vi "Create WebService.vi"() -> ()   [LabVIEW 2019, in "HTTP Server.lvlib"]
uses:
  HTTP Server.lvlib
  WebService reference.ctl
  Listener Information.ctl
panel:
  in  "WebService引用":T1={"IP Address"="127.0.0.1", "Port"=8003, "listener ID"=refnum}
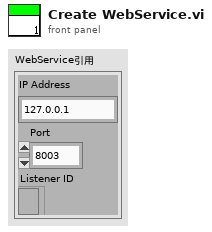
[diagram p1: front panel]
types:
  T1 = typedef "HTTP Server.lvlib/WebService reference.ctl" = cluster{"IP Address":string, "Port":u16, "listener ID":refnum<k5>}
  T2 = typedef "HTTP Server.lvlib/Listener Information.ctl" = cluster{"连接ID":refnum<k5>}
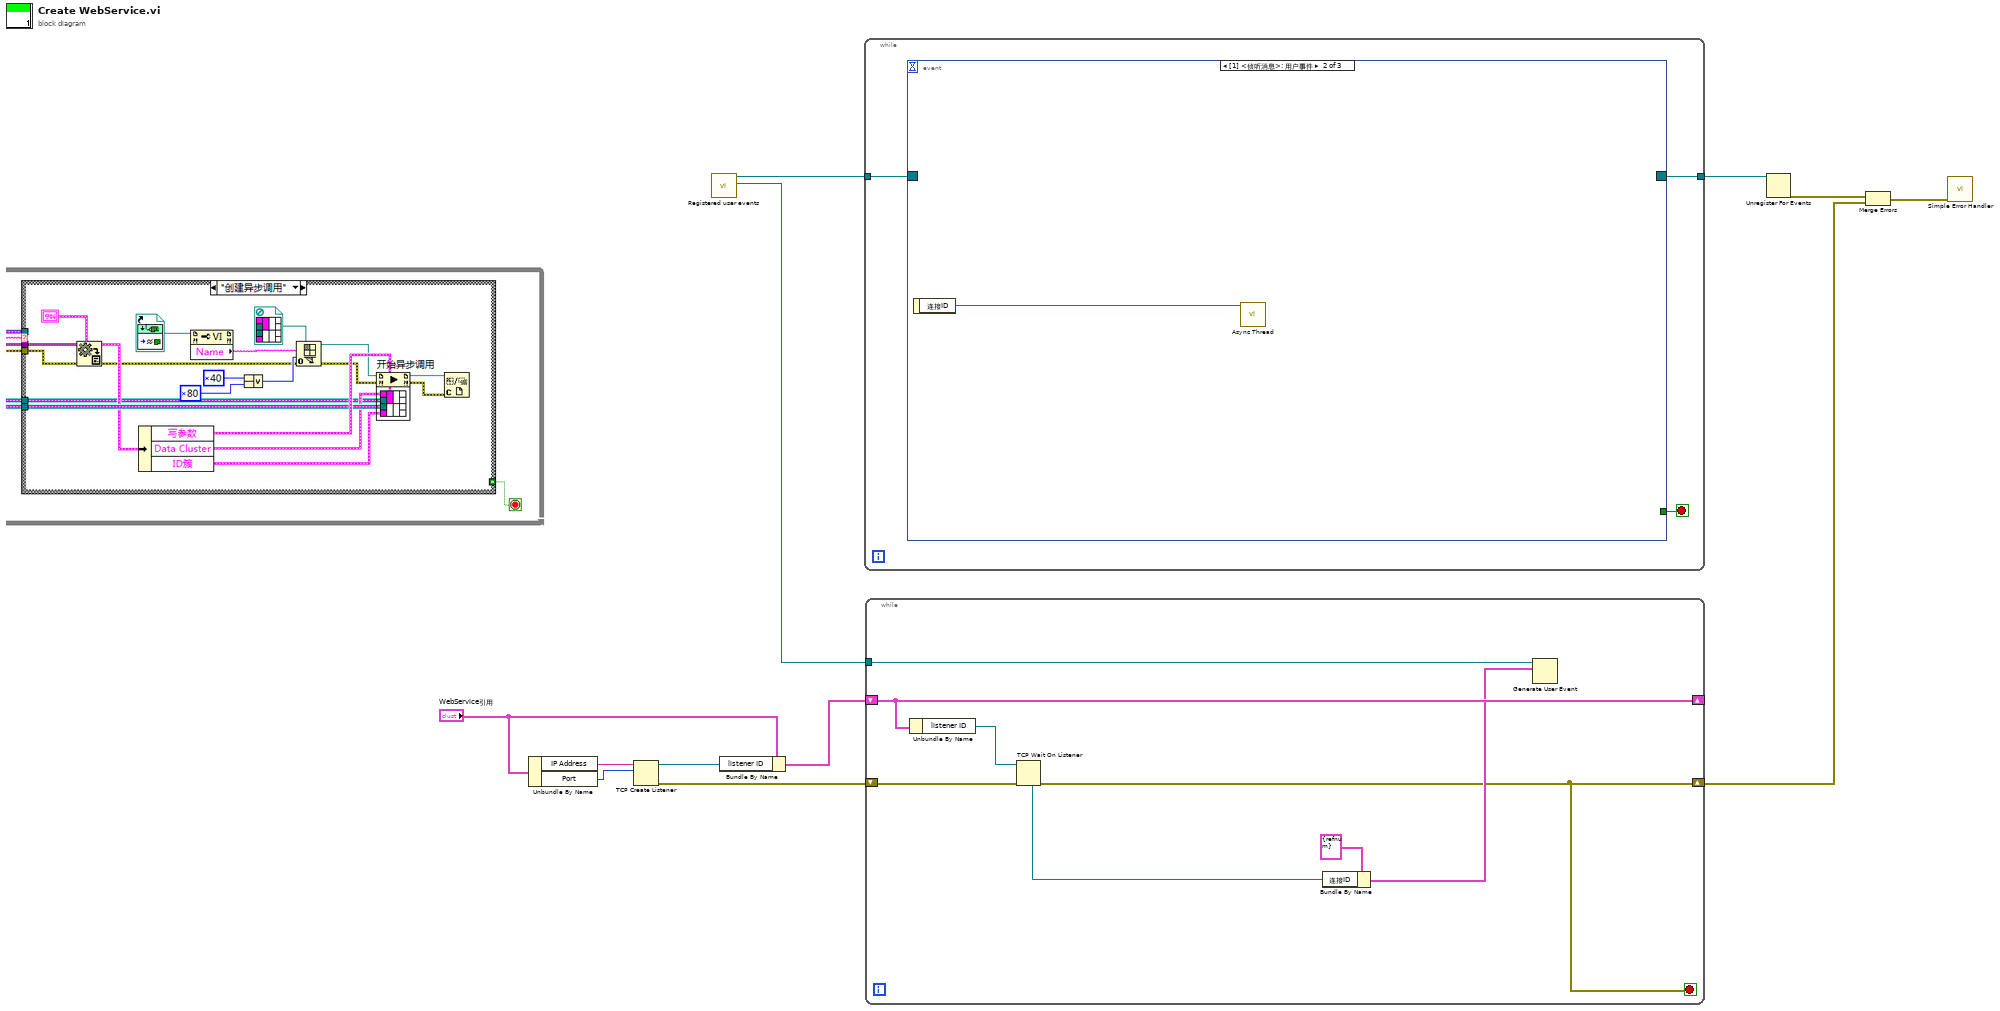
[diagram p0: block diagram]
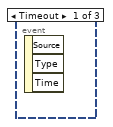
[diagram p2: hidden frame]
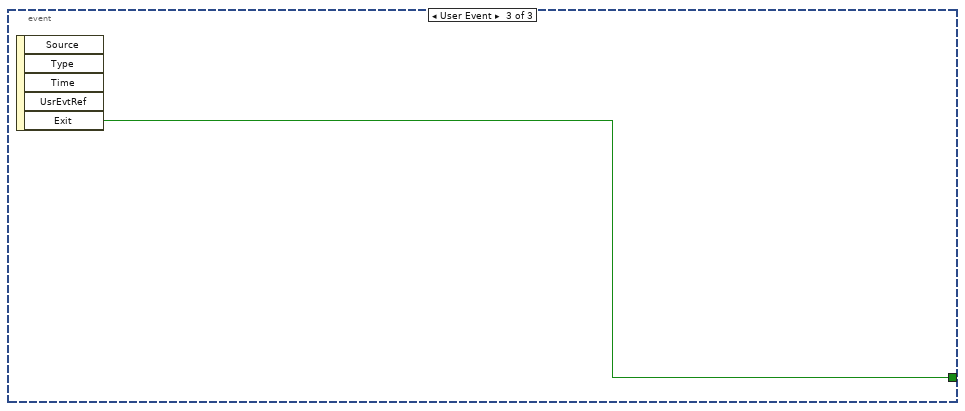
[diagram p3: hidden frame]
diagram:
  n1 = Unbundle By Name("WebService引用") -> ("IP Address"=w10:string, "Port"=w9:u16)
  n2 = TCP Create Listener(10:w9, 11:w10) -> (0:w5:errorcluster, 3:w7:refnum<k5>)  [unwired: 3 in, 1 out]
  n3 = call "Registered user events.vi"() -> ("用户事件输出_侦听消息"=w11:refnum<user-event>, "事件注册引用句柄"=w12:refnum<event-registration>)  [unwired: 9 in, 1 out]
  n4 = Bundle By Name(cluster="WebService引用", "listener ID"=w7) -> (w6:T1)
  n5 = while {
    tunnel: w12 -> [w15]
    tunnel: [w13] -> w4
    stop <- w14 stop-if-true
    n6 = event shown="[1] <侦听消息>: 用户事件" {
      selector: w15 -> [_ _ _]
      dyn-events: [_ _ _] -> w13
      timeout: _ -> [_ _ _]
      tunnel: [_ _ w17] -> w14
      event Timeout {
        n7 = event-data() -> ()  [unwired: 1 in, 3 out]
      }
      event User Event {
        n8 = event-data() -> ("连接ID"=w16:refnum<k5>)  [unwired: 1 in]
        n9 = call "Async Thread.vi"("TCP网络连接引用句柄"=w16) -> ()  [unwired: 11 in]
      }
      event User Event {
        n10 = event-data() -> ("Exit"=w17:bool)  [unwired: 1 in, 4 out]
      }
    }
  }
  n11 = while {
    tunnel: w11 -> [w25]
    shift-right: [w24] -> _
    shift-left: w6 -> [w24]
    shift-right: [w18] -> w2
    shift-left: w5 -> [w22]
    stop <- w18 stop-if-true
    n12 = Unbundle By Name(w24) -> ("listener ID"=w23:refnum<k5>)
    n13 = TCP Wait On Listener(8:w22, 11:w23) -> (0:w18:errorcluster, 4:w20:refnum<k5>)  [unwired: 2 in, 3 out]
    n14 = Bundle By Name(cluster=T2 {"连接ID"=refnum} ("事件数据"), "连接ID"=w20) -> (w19:T2)
    n15 = Generate User Event(user event=w25, event data cluster=w19) -> ()  [unwired: 2 in, 2 out]
  }
  n16 = Unregister For Events(event registration refnum=w4) -> (error out=w3:errorcluster)  [unwired: 1 in]
  n17 = Merge Errors(w3, w2) -> (w1:errorcluster)
  n18 = call <vilib>:"Simple Error Handler.vi"("error in (no error)"=w1) -> ()  [unwired: 4 in, 5 out]
